vi "LV Multiply (SubVI).vi"(10 "Array in":dbl[](array[numeric]), 11 "c":dbl) -> (3 "Array out":dbl[](array[numeric]))   [LabVIEW 2017]
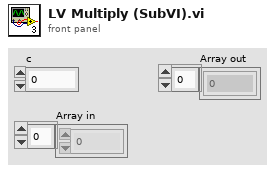
[diagram p1: front panel]
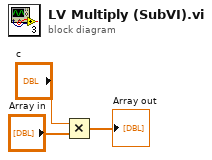
[diagram p0: block diagram]
diagram:
  n1 = Multiply(x="c", y="Array in") -> (x*y=→"Array out":dbl[])
